vi "Start Processs(static).vi"(8 "error in (no error)":errorcluster caption="错误输入（无错误）", 10 "fileName":string, 11 "ProcessClass 输入":refnum<class "ProcessClass.lvclass"> caption="DNL_LabVIEW Object in") -> (0 "error out":errorcluster caption="错误输出", 2 "Start":refnum<k24>, 3 "ProcessClass 输出":refnum<class "ProcessClass.lvclass"> caption="DNL_LabVIEW Object out")   [LabVIEW 2011, in "ProcessClass.lvclass"]
uses:
  ProcessClass.lvclass
  ProcessClass.lvclass/ProcessClass.ctl
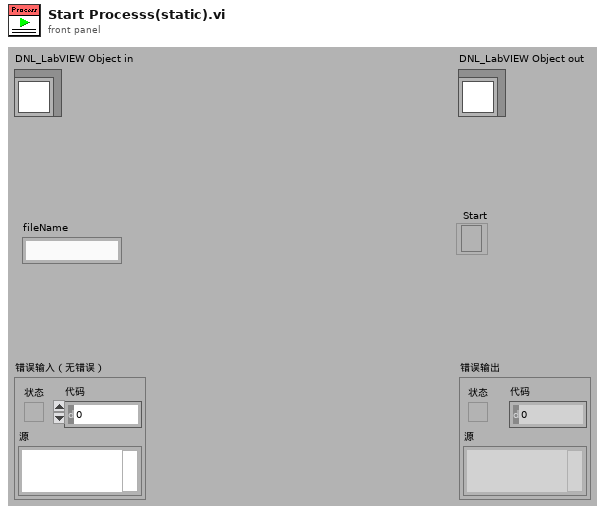
[diagram p1: front panel]
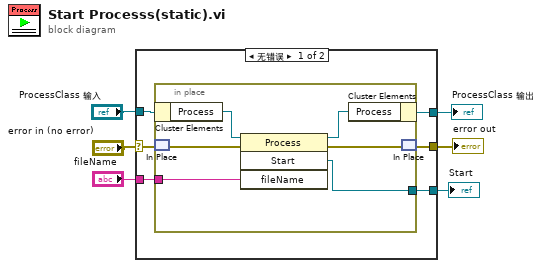
[diagram p0: block diagram]
diagram:
  n1 = case shown="无错误" "error in (no error)" {
    selector: "error in (no error)" -> [w12 w20]
    tunnel: [w11 w20] -> w5
    tunnel: [w7 w19] -> w3
    tunnel: "ProcessClass 输入" -> [w10 w19]
    tunnel: "fileName" -> [w9 _]
    tunnel: [w8 _] -> w1
    frame No Error {
      n2 = in-place {
        in-place-border: w9 -> [w16]
        in-place-border: [w15] -> w8
        n3 = in-place-cluster #1(w10) -> ("Process"=w18:refnum<k24>)
        n4 = in-place-match #2(w12) -> (w14:errorcluster)
        n5 = invoke class="Process" method="Start"(reference=w18, error in=w14, "fileName"=w16) -> (reference out=w17:refnum<k24>, error out=w13:errorcluster, "Start"=w15:refnum<k24>)  [unwired: 1 in, 1 out]
        n6 = in-place-cluster #1("Process"=w17) -> (w7:refnum<class "ProcessClass.lvclass">)
        n7 = in-place-match #2(w13) -> (w11:errorcluster)
      }
    }
    frame Error {
    }
  }
  "error out" <- w5
  "ProcessClass 输出" <- w3
  "Start" <- w1
